vi "Test Create HS256 JWT.vi"() -> ()   [LabVIEW 2017]
uses:
  JWT/JWT/JWT.lvclass
  JWT/Signature Algorithms.ctl
  JWT/JWT.lvlib
  JWT/JWT/Additional Standard Claims.ctl
panel:
  out "JWT":string
  in  "Key":string="@figbT|NKu|cn5P``Y!{gPpX3_e{bOe~"
  in  "Standard Claims":T1
  in  "JSON Payload":string="{\n  \"name\": \"John Smith\",\n  \"abilities\": [\"access\", \"test\"]\n}"
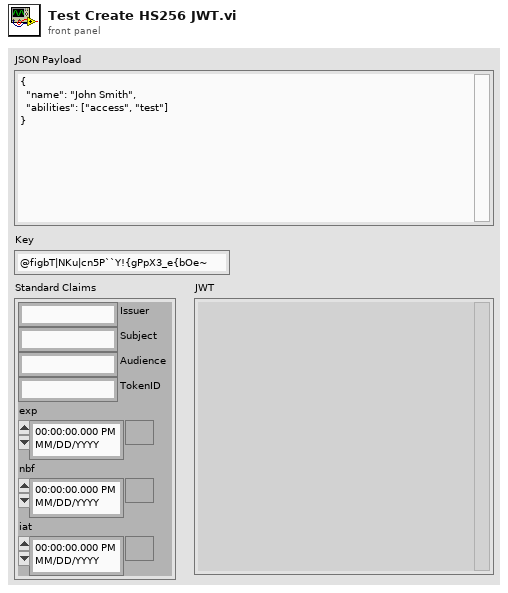
[diagram p1: front panel]
types:
  T1 = typedef "JWT.lvlib/JWT.lvclass/Additional Standard Claims.ctl" = cluster{"Issuer":string, "Subject":string, "Audience":string, "TokenID":string, "exp":timestamp, "nbf":timestamp, "iat":timestamp}
  T2 = typedef "JWT.lvlib/Signature Algorithms.ctl" = enum16{"none", "HS256"}
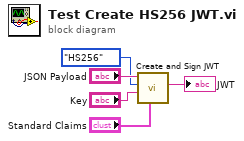
[diagram p0: block diagram]
diagram:
  n1 = call "Create and Sign JWT.vi"("Additional Standard Claims"="Standard Claims", "Key"="Key", "Signature Algorithm"=Signature_Algorithms."HS256", "JSON Payload"="JSON Payload") -> ("JWT"=→"JWT":string)  [unwired: 5 in, 2 out]
